vi "Vision Processing.vi"(4 "error in (no error)":errorcluster, 7 "Image Size":T2=enum."160x120") -> ()   [LabVIEW 2017]
doc: "This VI runs in parallel to other tasks. It gets images from the camera, processes them for color or shape and use that information to affect robot behavior."
uses:
  <vilib>/Rock Robotics/WPI/Camera/WPI_CameraImageSize.ctl
  <vilib>/Rock Robotics/WPI/Camera/WPI_CameraWhite Balance Values.ctl
  <vilib>/Rock Robotics/WPI/Camera/WPI_CameraExposure Values.ctl
  <vilib>/Rock Robotics/WPI/Camera/WPI_CameraFrameRate.ctl
  Robot Global Data.vi
  <vilib>/vision/NI_Vision_Development_Module.lvlib
panel:
  out "ParticleArea":dbl
  out "Map":T1
  in  "Lum":cluster{"Lower value":i32, "Upper value":i32}={"Lower value"=30, "Upper value"=100}
  in  "Sat":cluster{"Lower value":i32, "Upper value":i32}={"Lower value"=130, "Upper value"=255}
  in  "Hue":cluster{"Lower value":i32, "Upper value":i32}={"Lower value"=70, "Upper value"=130}
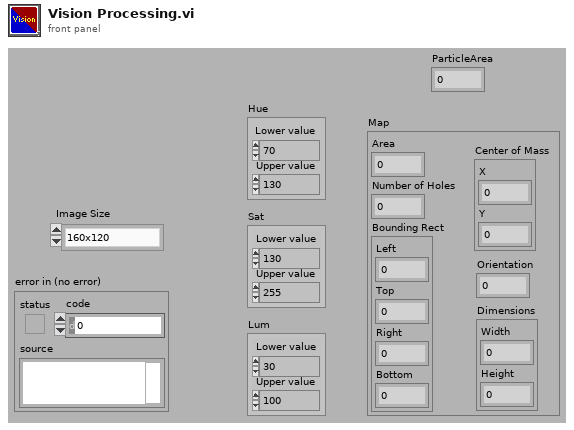
[diagram p1: front panel]
types:
  T1 = cluster{"Area":dbl, "Number of Holes":dbl, "Bounding Rect":cluster{"Left":dbl, "Top":dbl, "Right":dbl, "Bottom":dbl}, "Center of Mass":cluster{"X":dbl, "Y":dbl}, "Orientation":dbl, "Dimensions":cluster{"Width":dbl, "Height":dbl}}
  T2 = typedef "WPI_CameraImageSize.ctl" = enum16{"640x480", "320x240", "160x120", "Custom"}
  T3 = typedef "WPI_CameraFrameRate.ctl" = u32
  T4 = typedef "WPI_CameraExposure Values.ctl" = enum16{"Auto", "Flicker-free 50 Hz", "Flicker-free 60 Hz", "Hold current", "Custom"}
  T5 = typedef "WPI_CameraWhite Balance Values.ctl" = enum16{"Auto", "Fixed indoor", "Fixed outdoor 1", "Fixed outdoor 2", "Fixed fluorescent 1", "Fixed fluorescent 2", "Hold current", "Custom"}
  T6 = typedef "WPI_CameraDevRef.ctl" = cluster{"Camera Address":string, "CameraStatus":errorcluster}
  T7 = typedef "IMAQ Image.ctl" = refnum<image>
  T8 = typedef "Particle Parameters" = i32
  T9 = cluster{"Measurement Parameter":T8, "Range Lower Value":dbl, "Range Upper Value":dbl, "Range":bool, "Measurement Type":bool}[]
  T10 = typedef "Image Type" = u32
  T11 = cluster{"Area":dbl, "Number of Holes":dbl, "Bounding Rect":cluster{"Left":dbl, "Top":dbl, "Right":dbl, "Bottom":dbl}, "Center of Mass":cluster{"X":dbl, "Y":dbl}, "Orientation":dbl, "Dimensions":cluster{"Width":dbl, "Height":dbl}}[]
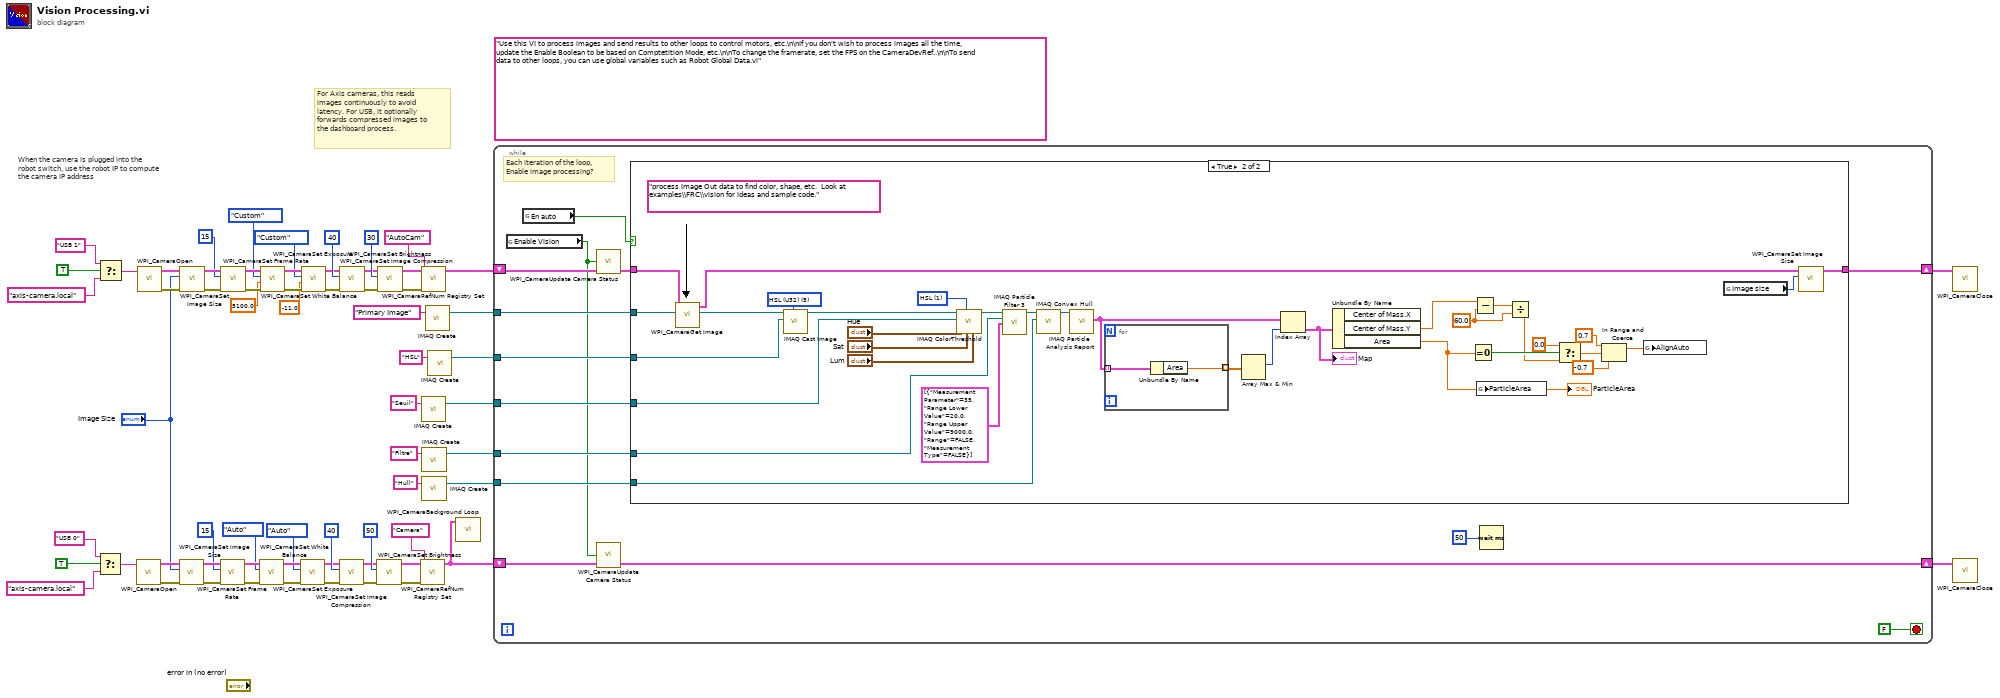
[diagram p0: block diagram]
diagram:
  (unwired) "Use this VI to process images and send results to other loops to control motors, etc.\n\nIf you don't wish to process images all the time, update the Enable Boolean to be based on Comptetition Mode, etc.\n\nTo change the framerate, set the FPS on the CameraDevRef..\n\nTo send data to other loops, you can use global variables such as Robot Global Data.vi"
  # "When the camera is plugged into the\nrobot switch, use the robot IP to compute\nthe camera IP address"
  # "For Axis cameras, this reads\nimages continuously to avoid\nlatency. For USB, it optionally\nforwards compressed images to\nthe dashboard process."
  n1 = Select(t="USB 0" ("format string"), s=TRUE ("dot notation? (F)"), f="axis-camera.local" ("format string")) -> (s? t:f=w6:string)
  n2 = Select(t="USB 1" ("format string"), s=TRUE ("dot notation? (F)"), f="axis-camera.local" ("format string")) -> (s? t:f=w39:string)
  n3 = call <vilib>:"WPI_CameraOpen.vi"("Camera Address"=w6) -> ("error out"=w18:errorcluster, "CameraDevRef"=w19:T6)  [unwired: 1 in, 8 out]
  n4 = call <vilib>:"WPI_CameraOpen.vi"("Camera Address"=w39) -> ("error out"=w54:errorcluster, "CameraDevRef"=w55:T6)  [unwired: 1 in, 8 out]
  n5 = call <vilib>:"WPI_CameraSet Image Size.vi"("error in (no error)"=w18, "Image Size"="Image Size", "CameraDevRef"=w19) -> ("error out"=w17:errorcluster, "CameraDevRef Out"=w20:T6)  [unwired: 1 in, 6 out]
  n6 = call <vilib>:"WPI_CameraSet Image Size.vi"("error in (no error)"=w54, "Image Size"="Image Size", "CameraDevRef"=w55) -> ("error out"=w53:errorcluster, "CameraDevRef Out"=w56:T6)  [unwired: 1 in, 6 out]
  n7 = call <vilib>:"WPI_CameraSet Frame Rate.vi"("error in (no error)"=w17, "Frame Rate (fps)"=T3 15, "CameraDevRef"=w20) -> ("error out"=w16:errorcluster, "CameraDevRef Out"=w22:T6)  [unwired: 7 out]
  n8 = call <vilib>:"WPI_CameraSet Frame Rate.vi"("error in (no error)"=w53, "Frame Rate (fps)"=T3 15, "CameraDevRef"=w56) -> ("error out"=w52:errorcluster, "CameraDevRef Out"=w58:T6)  [unwired: 7 out]
  n9 = call <vilib>:"WPI_CameraSet White Balance.vi"("error in (no error)"=w16, "White Balance"=WPI_CameraWhite_Balance_Values."Auto", "CameraDevRef"=w22) -> ("error out"=w15:errorcluster, "CameraDevRef Out"=w21:T6)  [unwired: 1 in, 6 out]
  n10 = call <vilib>:"WPI_CameraSet White Balance.vi"("error in (no error)"=w52, "Color Temp (K)"=5100.0, "White Balance"=WPI_CameraWhite_Balance_Values."Custom", "CameraDevRef"=w58) -> ("error out"=w51:errorcluster, "CameraDevRef Out"=w57:T6)  [unwired: 6 out]
  n11 = call <vilib>:"WPI_CameraSet Exposure.vi"("error in (no error)"=w15, "Exposure"=WPI_CameraExposure_Values."Auto", "CameraDevRef"=w21) -> ("error out"=w14:errorcluster, "CameraDevRef Out"=w24:T6)  [unwired: 1 in, 6 out]
  n12 = call <vilib>:"WPI_CameraSet Exposure.vi"("error in (no error)"=w51, "Exposure (%)"=-11.0, "Exposure"=WPI_CameraExposure_Values."Custom", "CameraDevRef"=w57) -> ("error out"=w50:errorcluster, "CameraDevRef Out"=w60:T6)  [unwired: 6 out]
  n13 = call <vilib>:"WPI_CameraSet Image Compression.vi"("error in (no error)"=w14, "Compression"=40, "CameraDevRef"=w24) -> ("error out"=w13:errorcluster, "CameraDevRef Out"=w23:T6)  [unwired: 7 out]
  n14 = call <vilib>:"WPI_CameraSet Image Compression.vi"("error in (no error)"=w50, "Compression"=40, "CameraDevRef"=w60) -> ("error out"=w49:errorcluster, "CameraDevRef Out"=w59:T6)  [unwired: 7 out]
  n15 = call <vilib>:"WPI_CameraSet Brightness.vi"("error in (no error)"=w13, "Brightness"=50, "CameraDevRef"=w23) -> ("error out"=w11:errorcluster, "CameraDevRef Out"=w12:T6)  [unwired: 1 in, 6 out]
  n16 = call <vilib>:"WPI_CameraSet Brightness.vi"("error in (no error)"=w49, "Brightness"=30, "CameraDevRef"=w59) -> ("error out"=w47:errorcluster, "CameraDevRef Out"=w48:T6)  [unwired: 1 in, 6 out]
  n17 = call <vilib>:"WPI_CameraRefNum Registry Set.vi"("error in (no error)"=w11, "refnum name"="Camera", "CameraDevRef"=w12) -> ("CameraDevRef"=w2:T6)  [unwired: 1 in, 7 out]
  n18 = call <vilib>:"WPI_CameraRefNum Registry Set.vi"("error in (no error)"=w47, "refnum name"="AutoCam", "CameraDevRef"=w48) -> ("CameraDevRef"=w43:T6)  [unwired: 1 in, 7 out]
  n19 = call "IMAQ Create"("Image Name"="Seuil") -> ("New Image"=w34:T7)  [unwired: 3 in, 2 out]
  n20 = call "IMAQ Create"("Image Name"="Filtre") -> ("New Image"=w32:T7)  [unwired: 3 in, 2 out]
  n21 = call "IMAQ Create"("Image Name"="Hull") -> ("New Image"=w30:T7)  [unwired: 3 in, 2 out]
  n22 = call "IMAQ Create"("Image Name"="Primary Image") -> ("New Image"=w64:T7)  [unwired: 3 in, 2 out]
  n23 = call "IMAQ Create"("Image Name"="HSL") -> ("New Image"=w36:T7)  [unwired: 3 in, 2 out]
  n24 = call <vilib>:"WPI_CameraBackground Loop.vi"("CameraDevRef"=w2) -> ()  [unwired: 11 in]
  n25 = while {
    shift-right: [w78] -> w42
    shift-left: w43 -> [w76]
    tunnel: w64 -> [w77]
    tunnel: w36 -> [w74]
    tunnel: w34 -> [w73]
    tunnel: w32 -> [w72]
    tunnel: w30 -> [w71]
    shift-right: [w68] -> w1
    shift-left: w2 -> [w70]
    stop <- FALSE stop-if-true
    # "Each iteration of the loop,\nEnable image processing?"
    n26 = global read "Robot Global Data.vi" "Enable Vision"() -> (w69:bool)
    n27 = global read "Robot Global Data.vi" "En auto"() -> (w66:bool)
    n28 = call <vilib>:"WPI_CameraUpdate Camera Status.vi"("CameraDevRef In"=w76, "Enable Vision"=w69) -> ("CameraDevRef Out"=w75:T6)  [unwired: 3 in]
    n29 = call <vilib>:"WPI_CameraUpdate Camera Status.vi"("CameraDevRef In"=w70, "Enable Vision"=w69) -> ("CameraDevRef Out"=w68:T6)  [unwired: 3 in]
    n30 = case shown="True" w66 {
      tunnel: w77 -> [_ w114]
      tunnel: [w80 w115] -> w78
      tunnel: w75 -> [w80 w93]
      tunnel: w74 -> [_ w97]
      tunnel: w73 -> [_ w96]
      tunnel: w72 -> [_ w94]
      tunnel: w71 -> [_ w95]
      frame False {
        # "If vision isn't started, keep loop\nfrom running full speed"
      }
      frame True {
        w90 = 60.0 ("y")
        w111 = u16 1 items=["RGB", "HSL", "HSV", "HSI"] ("Color Mode")
        w112 = T10 5 items=["Grayscale (U8)", "Grayscale (I16)", "Grayscale (SGL)", "Complex (CSG)", "RGB (U32)", "HSL (U32)", "RGB (U64)", "Grayscale (U16)"] ("Image Type")
        (unwired) "process Image Out data to find color, shape, etc.  Look at examples\\FRC\\vision for ideas and sample code."
        n31 = call <vilib>:"WPI_CameraGet Image.vi"("Image"=w114, "CameraDevRef"=w93) -> ("Image Out"=w98:T7, "CameraDevRef Out"=w92:T6)  [unwired: 1 in, 7 out]
        n32 = call "IMAQ Cast Image"("Image Type"=w112, "Image Dst"=w97, "Image Src"=w98) -> ("Image Dst Out"=w102:T7)  [unwired: 7 in, 1 out]
        n33 = call "IMAQ ColorThreshold"("Blue or Luma or Val or Inten Range"="Lum", "Green or Sat Range"="Sat", "Color Mode"=w111, "Red or Hue Range"="Hue", "Image Dst"=w96, "Image Src"=w102) -> ("Image Dst Out"=w107:T7)  [unwired: 4 in, 1 out]
        n34 = call "IMAQ Particle Filter 3"("Image Src"=w107, "Image Dst"=w94, "Selection Values"=T9 [{"Measurement Parameter"=35, "Range Lower Value"=20.0, "Range Upper Value"=9000.0, "Range"=FALSE, "Measurement Type"=FALSE}]) -> ("Image Dst Out"=w103:T7)  [unwired: 10 in, 2 out]
        n35 = call "IMAQ Convex Hull"("Image Dst"=w95, "Image Src"=w103) -> ("Image Dst Out"=w105:T7)  [unwired: 8 in, 1 out]
        n36 = call "IMAQ Particle Analysis Report"("Image"=w105) -> ("Particle Reports (Pixels)"=w100:T11)  [unwired: 5 in, 5 out]
        n37 = for {
          tunnel: w100 -> [w117] mode=indexing
          tunnel: [w116] -> w101 mode=indexing
          n38 = Unbundle By Name(w117) -> ("Area"=w116:dbl)
        }
        n39 = Array Max & Min(array=w101) -> (max index (indices)=w99:i32)  [unwired: 3 out]
        n40 = Index Array(array=w100, index=w99) -> (element=w104:T1)
        "Map" <- w104
        n41 = Unbundle By Name(w104) -> ("Center of Mass.Y"=w89:dbl, "Area"=w88:dbl)  [unwired: 1 out]
        "ParticleArea" <- w88
        n42 = Equal To 0?(x=w88) -> (x = 0?=w87:bool)
        n43 = Subtract(x=w89, y=w90) -> (x-y=w91:dbl)
        n44 = global write "Robot Global Data.vi" "ParticleArea"(w88) -> ()
        n45 = Divide(x=w91, y=w90) -> (x/y=w86:dbl)
        n46 = Select(t=0.0, s=w87, f=w86) -> (s? t:f=w84:dbl)
        n47 = In Range and Coerce(upper limit=0.7, x=w84, lower limit=-0.7) -> (coerced(x)=w83:dbl)  [unwired: 1 out]
        n48 = global write "Robot Global Data.vi" "AlignAuto"(w83) -> ()
        n49 = global read "Robot Global Data.vi" "image size"() -> (w113:T2)
        n50 = call <vilib>:"WPI_CameraSet Image Size.vi"("Image Size"=w113, "CameraDevRef"=w92) -> ("CameraDevRef Out"=w115:T6)  [unwired: 2 in, 7 out]
      }
    }
    n51 = Wait (ms)(milliseconds to wait=u32 50) -> ()  [unwired: 1 out]
  }
  n52 = call <vilib>:"WPI_CameraClose.vi"("CameraDevRef"=w42) -> ()  [unwired: 1 in, 10 out]
  n53 = call <vilib>:"WPI_CameraClose.vi"("CameraDevRef"=w1) -> ()  [unwired: 1 in, 10 out]
